vi "debug_PSF_Image.vi"() -> ()   [LabVIEW 2011]
panel:
  out "Focal Plane Scanner":dbl[][](graph)
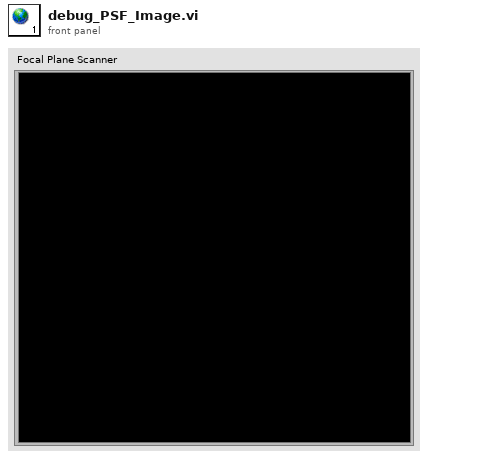
[diagram p1: front panel]
diagram:
